vi "Update Sampling Rate.vi"(8 "error in (no error)":errorcluster, 10 "Timing Parameter":T1={"rate"=1000.0, "samples per channel"=1000, "sample mode"=10123} {"sample mode" items=["Finite Samples"=10178, "Continuous Samples"=10123, "Hardware Timed Single Point"=12522]; "rate" format="%0.2f"}, 11 "PXIe 6363 in":refnum<class "PXIe 6363.lvclass">) -> (0 "error out":errorcluster, 3 "PXIe 6363 out":refnum<class "PXIe 6363.lvclass">)   [LabVIEW 2021, in "DAQ Hardware.lvlib" / "PXIe 6363.lvclass"]
uses:
  PXIe 6363.lvclass
  Timing AI DAQ Setting.ctl
  PXIe 6363.lvclass/PXIe 6363.ctl
  <resource>/objmgr/daqmx.rc
  DAQ Hardware.lvlib
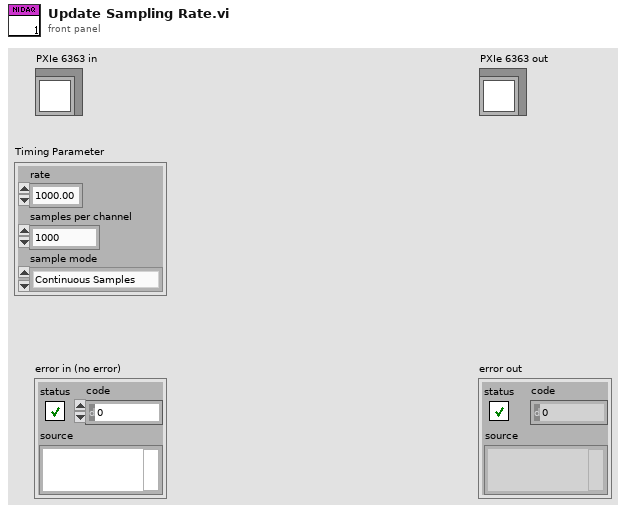
[diagram p1: front panel]
types:
  T1 = typedef "DAQ Hardware.lvlib/Timing AI DAQ Setting.ctl" = cluster{"rate":dbl, "samples per channel":i32, "sample mode":i32}
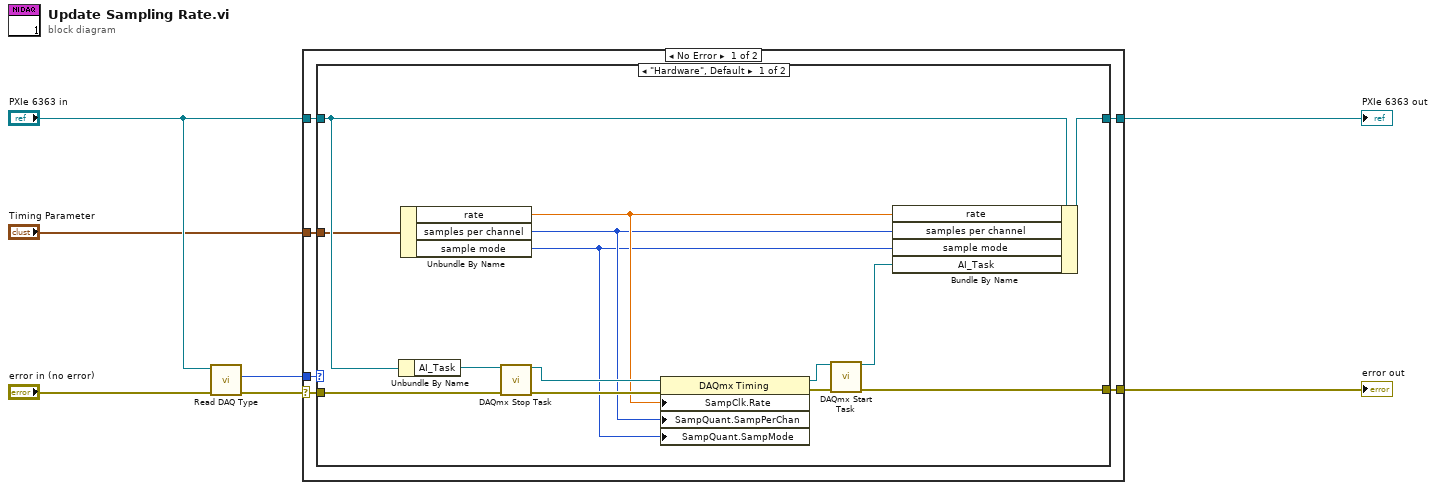
[diagram p0: block diagram]
diagram:
  n1 = call-dynamic "Read DAQ Type.vi"("error in (no error)"="error in (no error)", "PXIe 6363 in"="PXIe 6363 in") -> ("error out"=w6:errorcluster, "DAQ Type"=w5:enum16{"Hardware", "Simulation"})  [unwired: 7 in, 1 out]
  n2 = case shown="No Error" w6 {
    selector: w6 -> [w11 w30]
    tunnel: w5 -> [w13 _]
    tunnel: "PXIe 6363 in" -> [w12 w31]
    tunnel: [w10 w31] -> w3
    tunnel: [w9 w30] -> w2
    tunnel: "Timing Parameter" -> [w8 _]
    frame No Error {
      n3 = case shown="\"Hardware\", Default" w13 {
        tunnel: w12 -> [w27 w29]
        tunnel: w11 -> [w25 w28]
        tunnel: [w26 w29] -> w10
        tunnel: [w19 w28] -> w9
        tunnel: w8 -> [w17 _]
        frame "Hardware", Default {
          n4 = Unbundle By Name(w27) -> ("AI_Task"=w24:refnum<k21>)
          n5 = Unbundle By Name(w17) -> ("rate"=w16:dbl, "samples per channel"=w15:i32, "sample mode"=w14:i32)
          n6 = call <vilib>:"DAQmx Stop Task.vi"("task/channels in"=w24, "error in"=w25) -> ("task out"=w23:refnum<k21>, "error out"=w22:errorcluster)  [unwired: 12 in]
          n7 = property class="DAQmx Timing"(reference=w23, error in=w22, "SampClk.Rate"=w16, "SampQuant.SampPerChan"=w15, "SampQuant.SampMode"=w14) -> (reference out=w21:refnum<k21>, error out=w20:errorcluster)
          n8 = call <vilib>:"DAQmx Start Task.vi"("task/channels in"=w21, "error in"=w20) -> ("task out"=w18:refnum<k21>, "error out"=w19:errorcluster)  [unwired: 12 in]
          n9 = Bundle By Name(cluster=w27, "rate"=w16, "samples per channel"=w15, "sample mode"=w14, "AI_Task"=w18) -> (w26:refnum<class "PXIe 6363.lvclass">)
        }
        frame "Simulation" {
        }
      }
    }
    frame Error {
    }
  }
  "error out" <- w2
  "PXIe 6363 out" <- w3
